vi "ray_vector_to_array__v1.vi"(0 "x":ext, 1 "α":ext, 2 "y":ext, 3 "β":ext, 4 "z":ext, 5 "γ":ext) -> (14 "光線ベクトル":ext[][](array[numeric]))   [LabVIEW 2020]
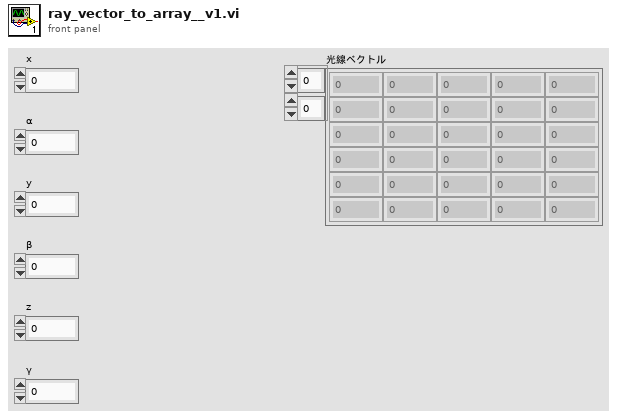
[diagram p1: front panel]
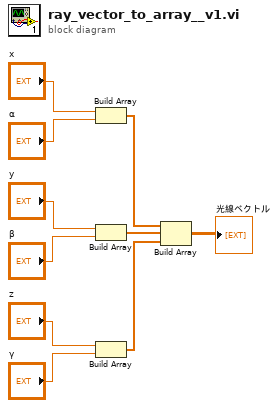
[diagram p0: block diagram]
diagram:
  n1 = Build Array("x", "α") -> (w2:ext[])
  n2 = Build Array("y", "β") -> (w4:ext[])
  n3 = Build Array("z", "γ") -> (w3:ext[])
  n4 = Build Array(w2, w4, w3) -> (→"光線ベクトル":ext[][])
